vi "TCP Send Operation.vi"(8 "error in":errorcluster) -> (0 "error out":errorcluster)   [LabVIEW 2013]
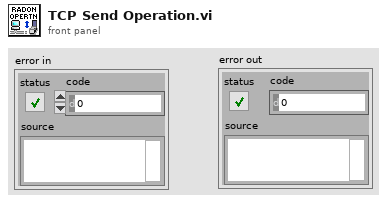
[diagram p1: front panel]
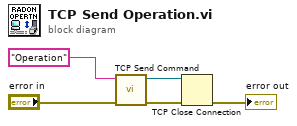
[diagram p0: block diagram]
diagram:
  n1 = call "TCP Send Command.vi"("error in"="error in", "Command"="Operation") -> ("error out"=w3:errorcluster, "connection ID out"=w1:refnum<k5>)  [unwired: 8 in]
  n2 = TCP Close Connection(connection ID=w1, error in (no error)=w3) -> (error out=→"error out":errorcluster)  [unwired: 1 in, 1 out]
